vi "Corss_Correlation (SubVI).vi"(10 "Array":dbl[](array[numeric]), 11 "Array 2":dbl[](array[numeric])) -> (1 "M":i32, 2 "Cross Corr. max value":dbl, 3 "Cross Corr":dbl[](graph), 4 "M-(N-1)":i32, 5 "N-1":i32)   [LabVIEW 2017]
uses:
  <vilib>/Analysis/NI_AALPro.lvlib
  <vilib>/Analysis/2dsp.llb/1D Cross Correlation (DBL).vi
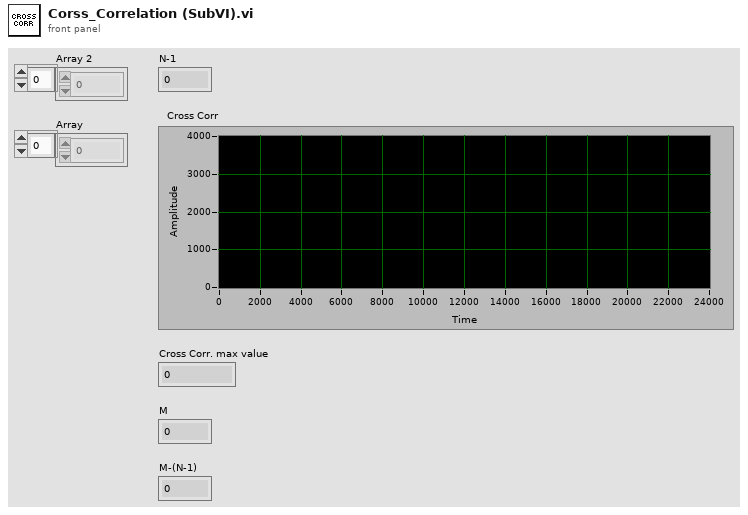
[diagram p1: front panel]
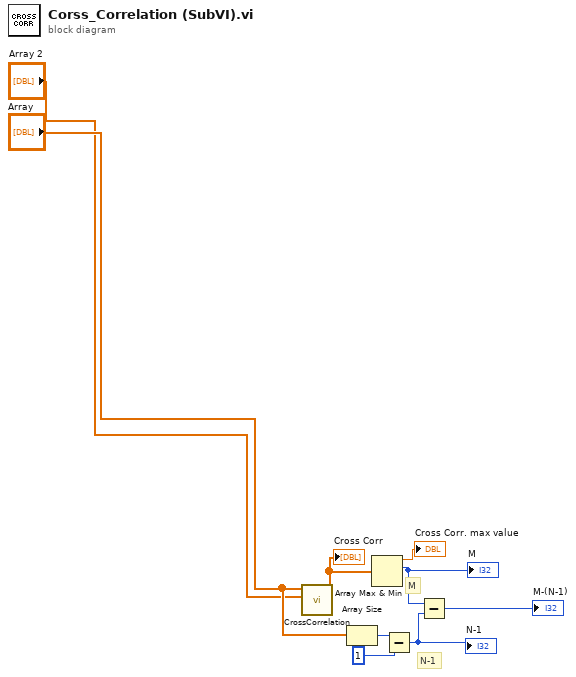
[diagram p0: block diagram]
diagram:
  # "N-1"
  # "M"
  n1 = call-poly <vilib>:"CrossCorrelation.vi"("Y"="Array 2", "X"="Array") -> ("Rxy"=w7:dbl[])  [unwired: 8 in, 1 out]
  "Cross Corr" <- w7
  n2 = Array Size(array="Array") -> (size(s)=w5:i32)
  n3 = Array Max & Min(array=w7) -> (max value=→"Cross Corr. max value":dbl, max index (indices)=w1:i32)  [unwired: 2 out]
  "M" <- w1
  n4 = Subtract(x=w5, y=1) -> (x-y=w3:i32)
  "N-1" <- w3
  n5 = Subtract(x=w1, y=w3) -> (x-y=→"M-(N-1)":i32)
